vi "Read initial setup.vi"(8 "error in (no error)":errorcluster, 11 "Channel in":refnum<class "Channel.lvclass">) -> (0 "error out":errorcluster, 3 "Channel out":refnum<class "Channel.lvclass">)   [LabVIEW 2018, in "Channel.lvclass"]
uses:
  Channel.lvclass
  Channel.lvclass/Channel.ctl
  <vilib>/Utility/config.llb/Read Key (Boolean).vi
  <vilib>/Utility/config.llb/Read Key (String).vi
  <vilib>/Utility/config.llb/NI_LVConfig.lvlib
panel:
  out "ACS configuration":T1
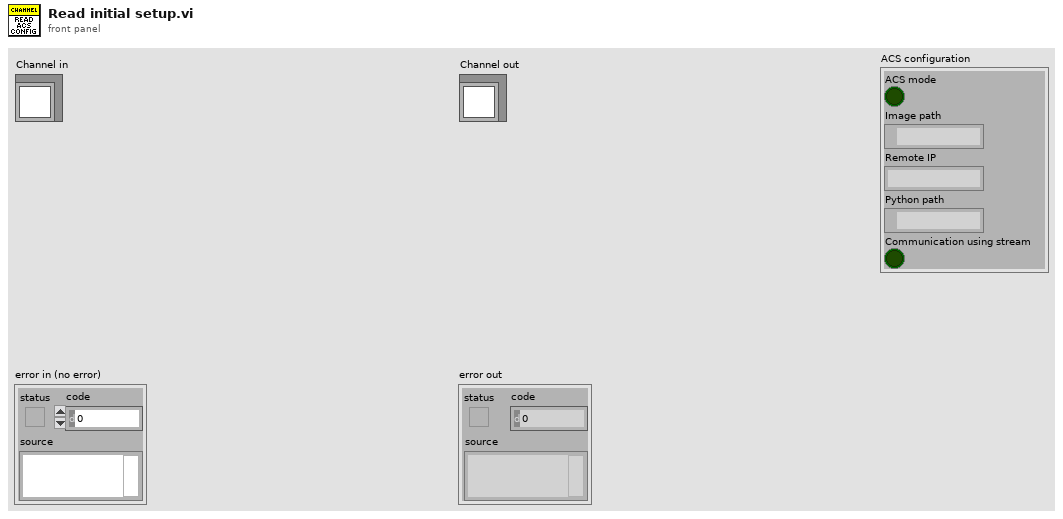
[diagram p1: front panel]
types:
  T1 = cluster{"ACS mode":bool, "Image path":path, "Remote IP":string, "Python path":path, "Communication using stream":bool}
  T2 = typedef "NI_LVConfig.lvlib/Config Data RefNum.ctl" = refnum<k1>
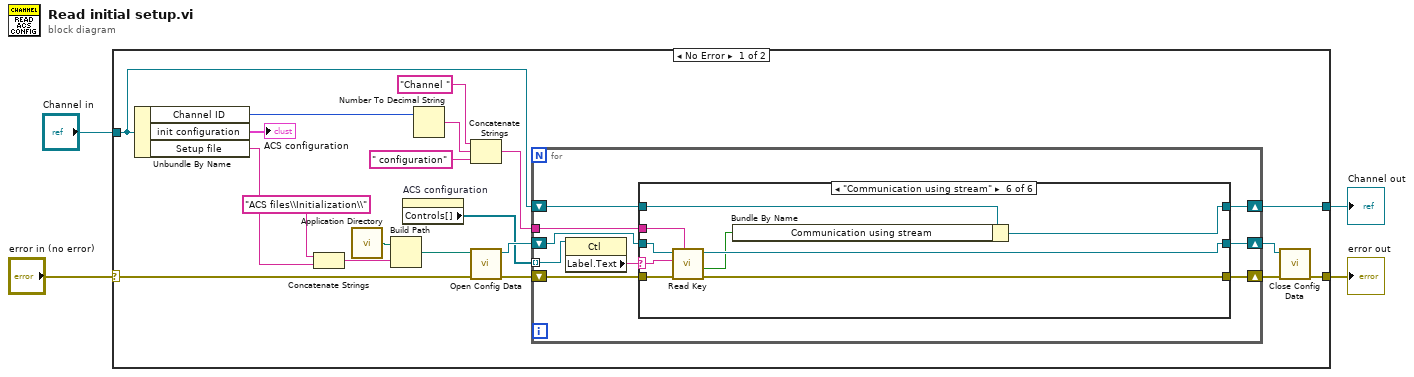
[diagram p0: block diagram]
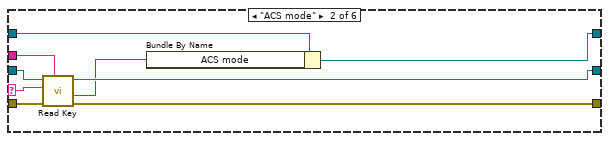
[diagram p3: hidden frame]
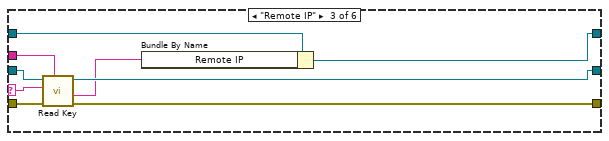
[diagram p4: hidden frame]
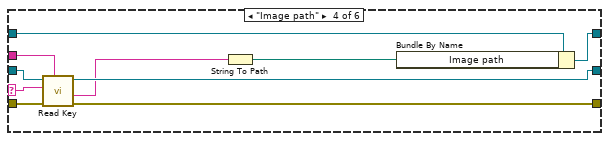
[diagram p5: hidden frame]
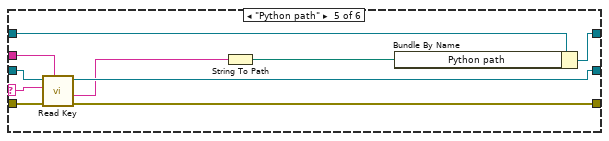
[diagram p6: hidden frame]
diagram:
  n1 = case shown="No Error" "error in (no error)" {
    selector: "error in (no error)" -> [w22 w85]
    tunnel: [w21 w85] -> w2
    tunnel: [w9 w84] -> w1
    tunnel: "Channel in" -> [w10 w84]
    frame No Error {
      n2 = Unbundle By Name(w10) -> ("Channel ID"=w5:u8, "init configuration"=→"ACS configuration":T1, "Setup file"=w8:string)
      n3 = Concatenate Strings("ACS files\\Initialization\\", w8) -> (w14:string)
      n4 = call <vilib>:"Application Directory.vi"() -> ("Application Directory"=w24:path)
      n5 = Build Path(base path=w24, name or relative path=w14) -> (appended path=w23:path)
      n6 = property on="ACS configuration" class="Clust (strict)"() -> ("Controls[]"=w6:refnum<vi>[])  [unwired: 2 in, 2 out]
      n7 = Number To Decimal String(number=w5) -> (decimal integer string=w16:string)  [unwired: 1 in]
      n8 = Concatenate Strings("Channel ", w16, " configuration") -> (w15:string)
      n9 = call <vilib>:"Open Config Data.vi"("error in (no error)"=w22, "configuration file path"=w23) -> ("error out"=w12:errorcluster, "refnum"=w18:T2)  [unwired: 7 in, 1 out]
      n10 = for {
        tunnel: w15 -> [w29]
        shift-right: [w32] -> w19
        shift-left: w18 -> [w33]
        shift-right: [w30] -> w20
        shift-left: w12 -> [w31]
        shift-right: [w27] -> w9
        shift-left: w10 -> [w28]
        tunnel: w6 -> [w26] mode=indexing
        n11 = property class="Ctl"(reference=w26) -> ("Label.Text"=w25:string)  [unwired: 1 in, 2 out]
        n12 = case shown="\"Communication using stream\"" w25 {
          selector: w25 -> [_ w40 w49 w59 w69 w78]
          tunnel: w33 -> [w36 w45 w54 w64 w74 w83]
          tunnel: [w36 w42 w51 w61 w71 w80] -> w32
          tunnel: w31 -> [w35 w44 w53 w63 w73 w82]
          tunnel: [w35 w43 w52 w62 w72 w81] -> w30
          tunnel: w29 -> [_ w41 w50 w60 w70 w79]
          tunnel: w28 -> [w34 w38 w47 w57 w67 w76]
          tunnel: [w34 w39 w48 w58 w68 w77] -> w27
          frame "False", Default {
          }
          frame "ACS mode" {
            n13 = call-poly <vilib>:"Read Key.vi"("section"=w41, "error in (no error)"=w44, "key"=w40, "refnum"=w45) -> ("error out"=w43:errorcluster, "value"=w37:bool, "refnum out"=w42:T2)  [unwired: 4 in, 1 out]
            n14 = Bundle By Name(cluster=w38, "ACS mode"=w37) -> (w39:refnum<class "Channel.lvclass">)
          }
          frame "Remote IP" {
            n15 = call-poly <vilib>:"Read Key.vi"("section"=w50, "error in (no error)"=w53, "key"=w49, "refnum"=w54) -> ("error out"=w52:errorcluster, "value"=w46:string, "refnum out"=w51:T2)  [unwired: 4 in, 1 out]
            n16 = Bundle By Name(cluster=w47, "Remote IP"=w46) -> (w48:refnum<class "Channel.lvclass">)
          }
          frame "Image path" {
            n17 = call-poly <vilib>:"Read Key.vi"("section"=w60, "error in (no error)"=w63, "key"=w59, "refnum"=w64) -> ("error out"=w62:errorcluster, "value"=w55:string, "refnum out"=w61:T2)  [unwired: 4 in, 1 out]
            n18 = String To Path(string=w55) -> (path=w56:path)
            n19 = Bundle By Name(cluster=w57, "Image path"=w56) -> (w58:refnum<class "Channel.lvclass">)
          }
          frame "Python path" {
            n20 = call-poly <vilib>:"Read Key.vi"("section"=w70, "error in (no error)"=w73, "key"=w69, "refnum"=w74) -> ("error out"=w72:errorcluster, "value"=w65:string, "refnum out"=w71:T2)  [unwired: 4 in, 1 out]
            n21 = String To Path(string=w65) -> (path=w66:path)
            n22 = Bundle By Name(cluster=w67, "Python path"=w66) -> (w68:refnum<class "Channel.lvclass">)
          }
          frame "Communication using stream" {
            n23 = call-poly <vilib>:"Read Key.vi"("section"=w79, "error in (no error)"=w82, "key"=w78, "refnum"=w83) -> ("error out"=w81:errorcluster, "value"=w75:bool, "refnum out"=w80:T2)  [unwired: 4 in, 1 out]
            n24 = Bundle By Name(cluster=w76, "Communication using stream"=w75) -> (w77:refnum<class "Channel.lvclass">)
          }
        }
      }
      n25 = call <vilib>:"Close Config Data.vi"("error in (no error)"=w20, "refnum"=w19) -> ("error out"=w21:errorcluster)  [unwired: 8 in, 1 out]
    }
    frame Error {
    }
  }
  "error out" <- w2
  "Channel out" <- w1
